vi "3.1.vi"(11 "Action":enum16{"Initialize", "Get Elapsed Time"}(ring)) -> (2 "Elapsed Time":dbl)   [LabVIEW 2013]
doc: "This VI is a Function Global Variable for Elapsed time with a custom format."
panel:
  out "fib(n)":i32
  in  "n":i16
  # "Overview: This VI is a FGV that acts as Elapsed time with a custom format.\nRequirements:\nLabVIEW 2012 (or compatible)\nInstructions:\n1. Run this VI.\n2. Try Get Elapsed time several times."
  # "The output format is MM.SS.\nFor example:\n1.10 is 1 Minute 10 Seconds\n0.56 is 0 Minutes 56 Seconds"
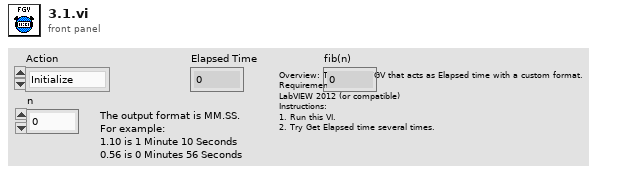
[diagram p1: front panel]
types:
  T1 = typedef "LVDateTimeRec.ctl" = cluster{"fractional second":dbl, "second":i32, "minute":i32, "hour":i32, "day of month":i32, "month":i32, "year":i32, "day of week":i32, "day of year":i32, "DST":i32}
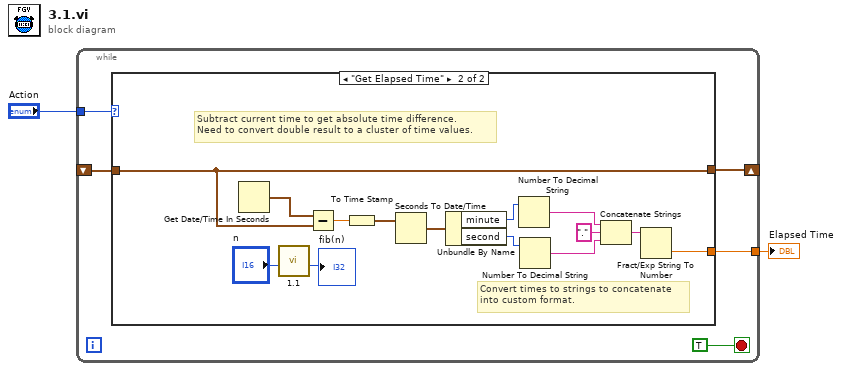
[diagram p0: block diagram]
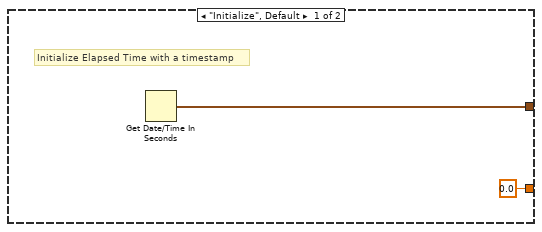
[diagram p2: hidden frame]
diagram:
  n1 = while {
    tunnel: "Action" -> [w6]
    shift-right: [w5] -> _
    shift-left: _ -> [w4]
    tunnel: [w3] -> w1
    stop <- TRUE stop-if-true
    n2 = case shown="\"Get Elapsed Time\"" w6 {
      tunnel: [w9 w21] -> w5
      tunnel: w4 -> [_ w21]
      tunnel: [0.0 w12] -> w3
      frame "Initialize", Default {
        # "Initialize Elapsed Time with a timestamp"
        n3 = Get Date/Time In Seconds() -> (seconds since 1Jan1904=w9:timestamp)
      }
      frame "Get Elapsed Time" {
        # "Convert times to strings to concatenate\ninto custom format."
        # "Subtract current time to get absolute time difference.\nNeed to convert double result to a cluster of time values."
        n4 = Get Date/Time In Seconds() -> (seconds since 1Jan1904=w23:timestamp)
        n5 = call "1.1.vi"("n"="n") -> ("fib(n)"=→"fib(n)":i32)  [unwired: 10 in]
        n6 = Subtract(x=w23, y=w21) -> (x-y=w22:dbl)
        n7 = To Time Stamp(1:w22) -> (0:w20:timestamp)
        n8 = Seconds To Date/Time(time stamp (now)=w20) -> (date time rec=w19:T1)  [unwired: 1 in]
        n9 = Unbundle By Name(w19) -> ("minute"=w17:i32, "second"=w18:i32)
        n10 = Number To Decimal String(number=w17) -> (decimal integer string=w15:string)  [unwired: 1 in]
        n11 = Number To Decimal String(number=w18) -> (decimal integer string=w14:string)  [unwired: 1 in]
        n12 = Concatenate Strings(w15, "." ("string"), w14) -> (w13:string)
        n13 = Fract/Exp String To Number(string=w13) -> (number=w12:dbl)  [unwired: 3 in, 1 out]
      }
    }
  }
  "Elapsed Time" <- w1
